vi "iconName.get.vi"(8 "error in (no error)":errorcluster, 11 "type in":refnum<class "type.lvclass">) -> (0 "error out":errorcluster, 2 "iconName":string, 3 "type out":refnum<class "type.lvclass">)   [LabVIEW 2020, in "type.lvclass"]
uses:
  type.lvclass
  type.lvclass/type.ctl
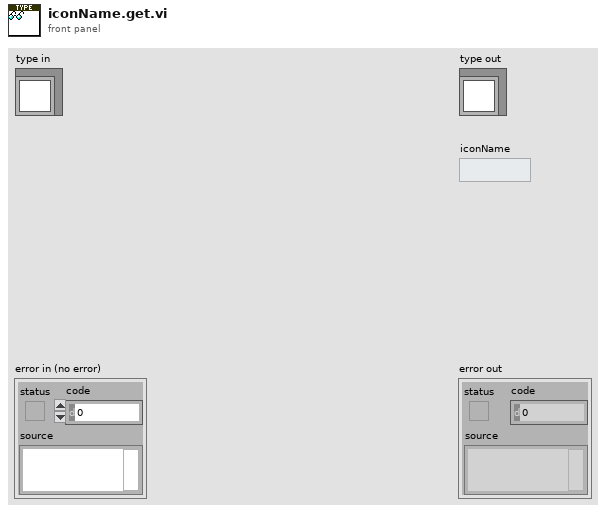
[diagram p1: front panel]
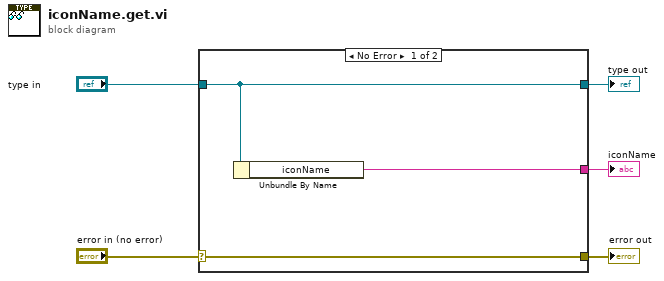
[diagram p0: block diagram]
diagram:
  n1 = case shown="No Error" "error in (no error)" {
    selector: "error in (no error)" -> [w8 w9]
    tunnel: [w8 w9] -> w4
    tunnel: [w7 w10] -> w2
    tunnel: "type in" -> [w7 w10]
    tunnel: [w6 _] -> w1
    frame No Error {
      n2 = Unbundle By Name(w7) -> ("iconName"=w6:string)
    }
    frame Error {
    }
  }
  "error out" <- w4
  "type out" <- w2
  "iconName" <- w1
